vi "Calculate Histogram from ADC Values.vi"(7 "Switch X/Y":bool, 11 "Values":cluster{"ADC Values":i32[]}[](array[cluster])) -> (3 "Histogram Data":cluster{cluster{dbl, dbl}[]}[](array[cluster]))   [LabVIEW 2019, in "Muon Data Post-Processing.lvlib"]
uses:
  <vilib>/Utility/miscctls.llb/LVMapReplaceAction.ctl
  <vilib>/Analysis/1siggen.llb/Ramp Pattern by Delta.vi
  Muon Data Post-Processing.lvlib
  <vilib>/Analysis/NI_AALBase.lvlib
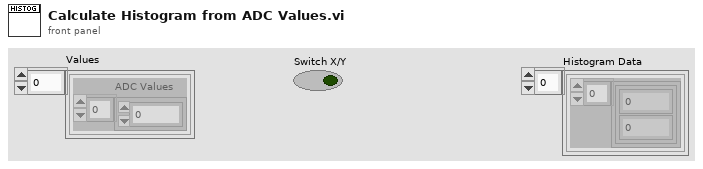
[diagram p1: front panel]
types:
  T1 = typedef "LVMapReplaceAction.ctl" = enum32{"Modify Entry only if found", "Add or Modify Entry", "Delete Entry"}
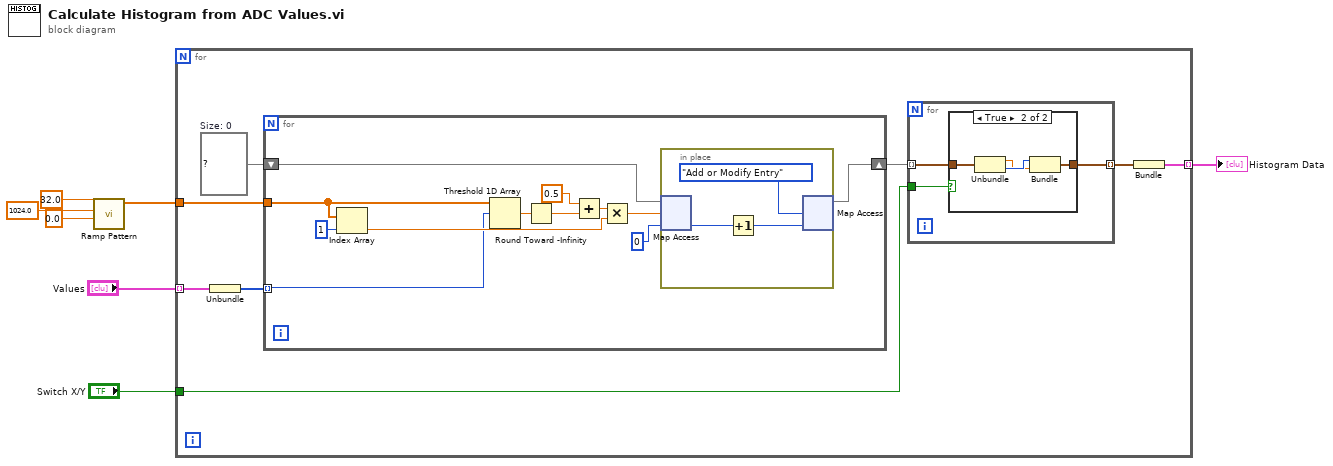
[diagram p0: block diagram]
diagram:
  n1 = call-poly <vilib>:"Ramp Pattern.vi"("start"=0.0, "end"=1024.0, "delta"=32.0) -> ("Ramp Pattern"=w4:dbl[])  [unwired: 6 in, 2 out]
  n2 = for {
    tunnel: w4 -> [w15]
    tunnel: [w9] -> w3 mode=indexing
    tunnel: "Switch X/Y" -> [w12]
    tunnel: "Values" -> [w10] mode=indexing
    w14 = map{dbl, i32} {}  # Size: 0
    n3 = Unbundle(w10) -> ("ADC Values"=w11:i32[])
    n4 = for {
      tunnel: w11 -> [w24] mode=indexing
      shift-right: [w27] -> w13
      shift-left: w14 -> [w26]
      tunnel: w15 -> [w25]
      n5 = Index Array(array=w25, index=1) -> (element=w35:dbl)
      n6 = Threshold 1D Array(2:w24, 3:w25) -> (0:w34:dbl)  [unwired: 1 in]
      n7 = Round Toward -Infinity(1:w34) -> (0:w33:dbl)
      n8 = Add(x=0.5, y=w33) -> (x+y=w32:dbl)
      n9 = Multiply(x=w32, y=w35) -> (x*y=w29:dbl)
      n10 = in-place {
        n11 = in-place-map #1(w26, w29, 0) -> (w38:i32)  [unwired: 1 out]
        n12 = Increment(x=w38) -> (x+1=w37:i32)
        n13 = in-place-map #1(w37, LVMapReplaceAction."Add or Modify Entry" ("action")) -> (w27:map{dbl, i32})  [unwired: 2 out]
      }
    }
    n14 = for {
      tunnel: w13 -> [w17] mode=indexing
      tunnel: [w18] -> w8 mode=indexing
      tunnel: w12 -> [w16]
      n15 = case shown="True" w16 {
        tunnel: [w19 w20] -> w18
        tunnel: w17 -> [w19 w23]
        frame False {
        }
        frame True {
          n16 = Unbundle(w23) -> (w21:dbl, w22:i32)
          n17 = Bundle(w22, w21) -> (w20:cluster{i32, dbl})  [unwired: 1 in]
        }
      }
    }
    n18 = Bundle(w8) -> (w9:cluster{cluster{dbl, dbl}[]})  [unwired: 1 in]
  }
  "Histogram Data" <- w3
